vi "setUp.vi"(8 "error in (no error)":errorcluster, 11 "reference in":refnum<class "Bus Controller Suite.lvclass">) -> (0 "error out":errorcluster, 3 "reference out":refnum<class "Bus Controller Suite.lvclass">)   [LabVIEW 2016, in "Bus Controller Suite.lvclass"]
doc: "setUp runs prior to the test method during test execution. Use this method to initialize any object data required by your tests."
uses:
  Bus Controller Suite.lvclass
  <vilib>/addons/_JKI Toolkits/VI Tester/TestSuite.llb/TestSuite.lvclass
  1553 Test/1553 Test.lvclass
  D:/Program Files (x86)/National Instruments/LabVIEW 2016/vi.lib/addons/_JKI Toolkits/VI Tester/TestCase.llb/TestCase.lvclass
  D:/Program Files (x86)/National Instruments/LabVIEW 2016/vi.lib/addons/_JKI Toolkits/VI Tester/TestSuite.llb/TestSuite.lvclass
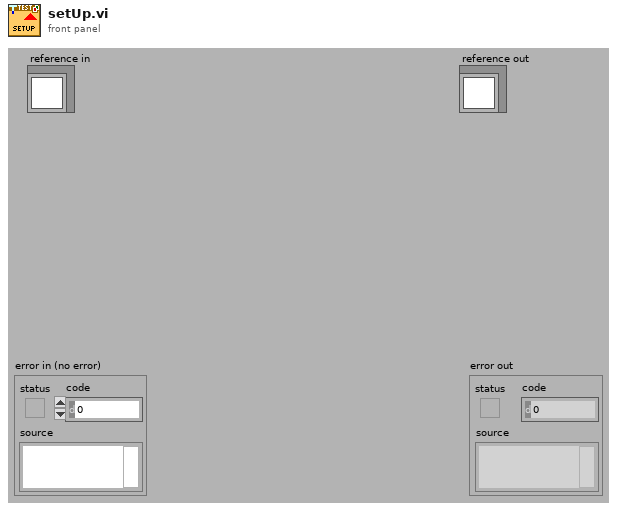
[diagram p1: front panel]
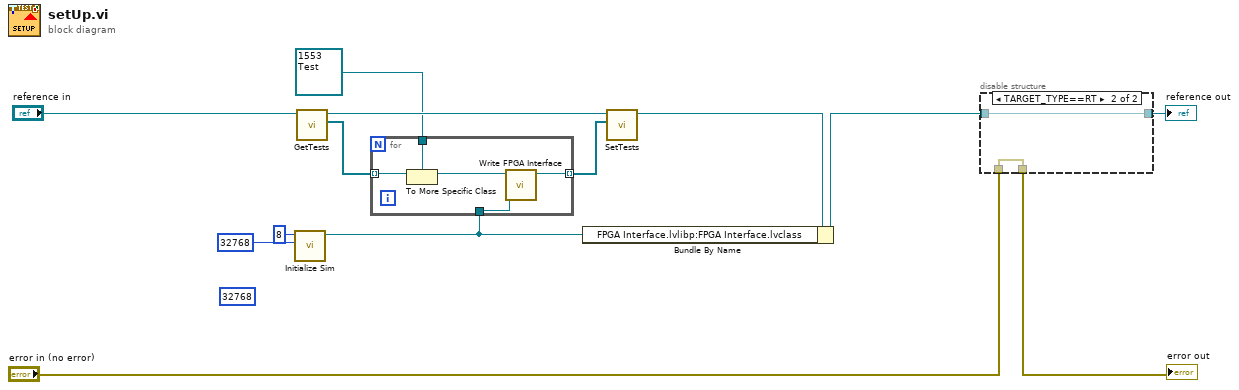
[diagram p0: block diagram]
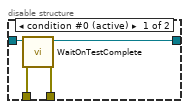
[diagram p2: hidden frame]
diagram:
  (unwired) 32768 ("Memory Size (32k)")
  n1 = call "Initialize Sim.vi"("Memory Size (32k)"=32768, "Components (8)"=8) -> ("FPGA Sim out"=w3:refnum<class "FPGA Sim.lvclass">)  [unwired: 8 in, 1 out]
  n2 = call-dynamic "GetTests.vi"("TestSuite in"="reference in") -> ("tests"=w6:refnum<class>[], "TestSuite in"=w8:refnum<class "Bus Controller Suite.lvclass">)  [unwired: 8 in, 1 out]
  n3 = for {
    tunnel: w6 -> [w18] mode=indexing
    tunnel: refnum<class "1553 Test.lvclass"> refnum ("1553 Test.lvclass") -> [w17]
    tunnel: [w15] -> w4 mode=indexing
    tunnel: w3 -> [w14]
    n4 = To More Specific Class(target class=w17, reference=w18) -> (specific class reference=w16:refnum<class "1553 Test.lvclass">)  [unwired: 1 in, 1 out]
    n5 = call-dynamic "Write FPGA Interface.vi"("FPGA Interface"=w14, "1553 Test in"=w16) -> ("1553 Test out"=w15:refnum<class "1553 Test.lvclass">)  [unwired: 8 in, 1 out]
  }
  n6 = call-dynamic "SetTests.vi"("tests"=w4, "TestSuite in"=w8) -> ("TestSuite in"=w7:refnum<class "Bus Controller Suite.lvclass">)  [unwired: 8 in, 1 out]
  n7 = Bundle By Name(cluster=w7, "FPGA Interface.lvlibp:FPGA Interface.lvclass"=w3) -> (w1:refnum<class "Bus Controller Suite.lvclass">)
  n8 = disable-structure shown="TARGET_TYPE==RT" {
    disable-tunnel: w1 -> [w22 w23]
    disable-tunnel: [w21 w23] -> w13
    disable-tunnel: "error in (no error)" -> [w20 w24]
    disable-tunnel: [w19 w24] -> w11
    frame condition #0 (active) {
      n9 = call <vilib>:"WaitOnTestComplete.vi"("error in (no error)"=w20, "TestSuite in"=w22) -> ("error out"=w19:errorcluster, "TestSuite out"=w21:refnum<class "Bus Controller Suite.lvclass">)  [unwired: 8 in]
    }
    frame condition #1 {
    }
  }
  "error out" <- w11
  "reference out" <- w13
